vi "PZT open channal.vi"(2 "error in (no error)":errorcluster caption="错误输入（无错误）", 3 "通道":i32, 4 "VISA resource name":refnum<visa-resource-name> caption="VISA资源名称") -> (0 "错误输出":errorcluster, 1 "VISA资源名称输出":refnum<visa-resource-name>)   [LabVIEW 2019]
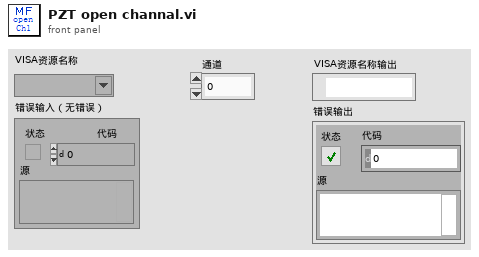
[diagram p1: front panel]
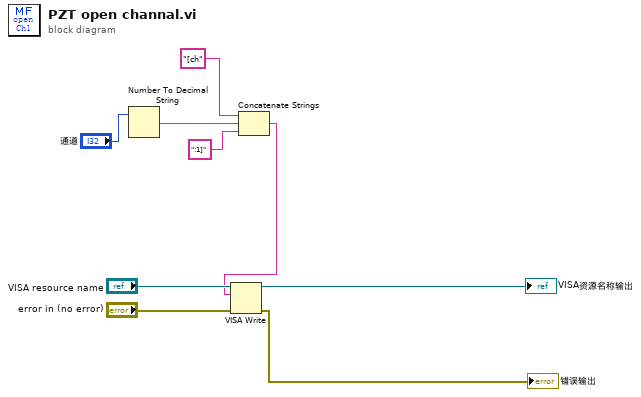
[diagram p0: block diagram]
diagram:
  n1 = Number To Decimal String(number="通道") -> (decimal integer string=w3:string)  [unwired: 1 in]
  n2 = Concatenate Strings("[ch" ("字符串"), w3, ":1]" ("字符串")) -> (w5:string)
  n3 = VISA Write(VISA resource name="VISA resource name", write buffer=w5, error in (no error)="error in (no error)") -> (VISA resource name out=→"VISA资源名称输出":refnum<visa-resource-name>, error out=→"错误输出":errorcluster)  [unwired: 1 out]
